vi "Demo 1 - FGEN and MSO.vi"() -> ()   [LabVIEW 2017]
uses:
  <vilib>/VirtualBench/_MSO Configure Timing6.vi
  <vilib>/VirtualBench/_FGEN Configure Standard Waveform0.vi
  <vilib>/VirtualBench/VirtualBench.lvlib
panel:
  in  "Frequency":dbl(knob) scale=0.0..10000.0
  in  "VirtualBench Device IO Control":tag
  out "Signal Plot":waveform(dbl)[](graph)
  in  "stop":bool
  in  "DC Offset":dbl caption="DC Offset (no change)"
  in  "Amplitude":dbl(slide)=2.0 caption="Amplitude (no change)" scale=0.0..10.0
  in  "Waveform Function":i32(ring) caption="Waveform Function (no change)" items=["Sine", "Square", "Triangle/Ramp", "DC"]
  in  "Duty Cycle":dbl=50.0 caption="Duty Cycle (no change)"
  # "Waveform Settings"
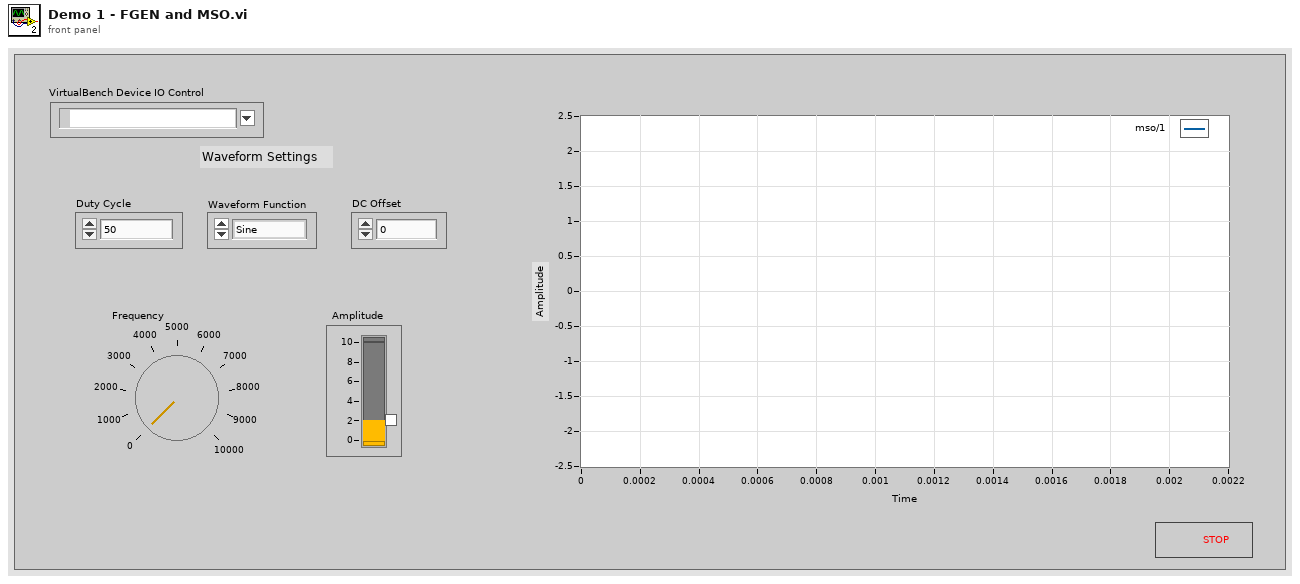
[diagram p1: front panel]
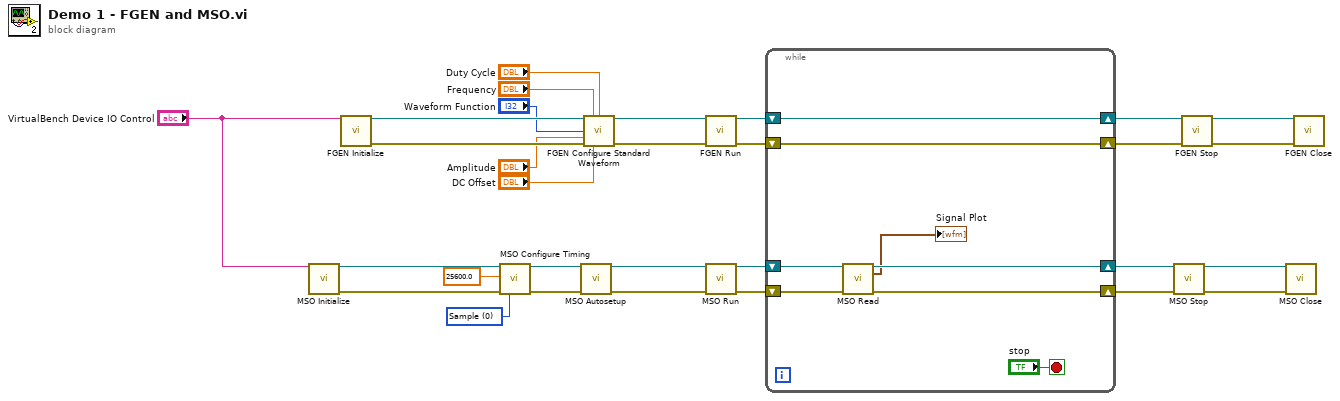
[diagram p0: block diagram]
diagram:
  w3 = 0 items=["Sample", "Peak Detect"] ("Sampling Mode")
  n1 = call <vilib>:"MSO Initialize.vi"("Device Name"="VirtualBench Device IO Control") -> ("Instrument Handle Out"=w6:refnum<k21>, "Error Out"=w19:errorcluster)  [unwired: 13 in]
  n2 = call <vilib>:"FGEN Initialize.vi"("Device Name"="VirtualBench Device IO Control") -> ("Instrument Handle Out"=w25:refnum<k21>, "Error Out"=w24:errorcluster)  [unwired: 13 in]
  n3 = call-poly <vilib>:"MSO Configure Timing.vi"("Instrument Handle In"=w6, "Sample Rate"=25600.0, "Error In"=w19, "Sampling Mode"=w3) -> ("Instrument Handle Out"=w5:refnum<k21>, "Error Out"=w7:errorcluster)  [unwired: 10 in]
  n4 = call <vilib>:"MSO Autosetup.vi"("Instrument Handle In"=w5, "Error In"=w7) -> ("Instrument Handle Out"=w18:refnum<k21>, "Error Out"=w17:errorcluster)  [unwired: 12 in]
  n5 = call-poly <vilib>:"FGEN Configure Standard Waveform.vi"("Instrument Handle In"=w25, "Frequency"="Frequency", "Duty Cycle"="Duty Cycle", "Waveform Function"="Waveform Function", "Amplitude"="Amplitude", "Error In"=w24, "DC Offset"="DC Offset") -> ("Instrument Handle Out"=w30:refnum<k21>, "Error Out"=w29:errorcluster)  [unwired: 7 in]
  n6 = call <vilib>:"FGEN Run.vi"("Instrument Handle In"=w30, "Error In"=w29) -> ("Instrument Handle Out"=w9:refnum<k21>, "Error Out"=w28:errorcluster)  [unwired: 12 in]
  n7 = call <vilib>:"MSO Run.vi"("Instrument Handle In"=w18, "Error In"=w17) -> ("Instrument Handle Out"=w16:refnum<k21>, "Error Out"=w15:errorcluster)  [unwired: 12 in]
  n8 = while {
    shift-right: [w33] -> w10
    shift-left: w28 -> [w33]
    shift-right: [w37] -> w14
    shift-left: w16 -> [w32]
    shift-right: [w36] -> w13
    shift-left: w15 -> [w38]
    shift-right: [w34] -> w8
    shift-left: w9 -> [w34]
    stop <- "stop" stop-if-true
    n9 = call <vilib>:"MSO Read.vi"("Instrument Handle In"=w32, "Error In"=w38) -> ("Instrument Handle Out"=w37:refnum<k21>, "Analog Waveforms"=→"Signal Plot":waveform(dbl)[], "Error Out"=w36:errorcluster)  [unwired: 8 in, 3 out]
  }
  n10 = call <vilib>:"MSO Stop.vi"("Instrument Handle In"=w14, "Error In"=w13) -> ("Instrument Handle Out"=w12:refnum<k21>, "Error Out"=w11:errorcluster)  [unwired: 12 in]
  n11 = call <vilib>:"FGEN Stop.vi"("Instrument Handle In"=w8, "Error In"=w10) -> ("Instrument Handle Out"=w27:refnum<k21>, "Error Out"=w26:errorcluster)  [unwired: 12 in]
  n12 = call <vilib>:"MSO Close.vi"("Instrument Handle In"=w12, "Error In"=w11) -> ()  [unwired: 13 in, 1 out]
  n13 = call <vilib>:"FGEN Close.vi"("Instrument Handle In"=w27, "Error In"=w26) -> ()  [unwired: 13 in, 1 out]
